vi "Write Database.vi"(8 "error in (no error)":errorcluster, 10 "Database.lvlib:Database":refnum<class "Database.lvclass">, 11 "Display in":refnum<class "Display.lvclass">) -> (0 "error out":errorcluster, 3 "Display out":refnum<class "Display.lvclass">)   [LabVIEW 2015, in "UserManagement.lvlib" / "Display.lvclass"]
uses:
  Display.lvclass
  DatabaseManagement/Database.lvclass
  Display.lvclass/Display.ctl
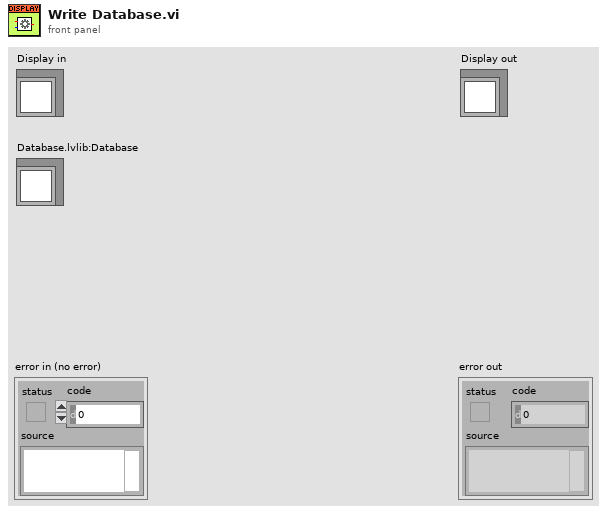
[diagram p1: front panel]
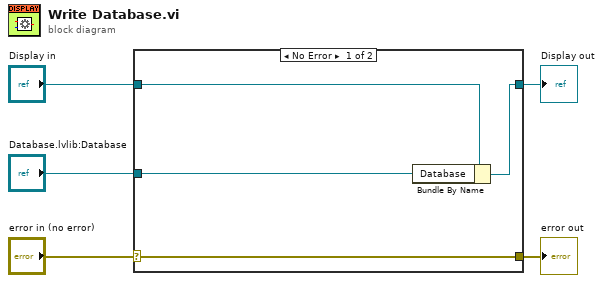
[diagram p0: block diagram]
diagram:
  n1 = case shown="No Error" "error in (no error)" {
    selector: "error in (no error)" -> [w9 w10]
    tunnel: [w9 w10] -> w4
    tunnel: [w7 w11] -> w2
    tunnel: "Display in" -> [w8 w11]
    tunnel: "Database.lvlib:Database" -> [w6 _]
    frame No Error {
      n2 = Bundle By Name(cluster=w8, "Database"=w6) -> (w7:refnum<class "Display.lvclass">)
    }
    frame Error {
    }
  }
  "error out" <- w4
  "Display out" <- w2
